vi "Value by Names.vi"(8 "error in (no error)":errorcluster, 10 "Children Names":string[](array[string]), 11 "OpenHW in":refnum<class "OpenHW.lvclass">) -> (0 "error out":errorcluster, 2 "HW Node":T1, 3 "OpenHW out":refnum<class "OpenHW.lvclass">)   [LabVIEW 2022 SP3, in "open-hw-mon-lv.lvlib" / "OpenHW.lvclass"]
uses:
  OpenHW.lvclass
  OpenHW.lvclass/OpenHW.ctl
  HW Node.ctl
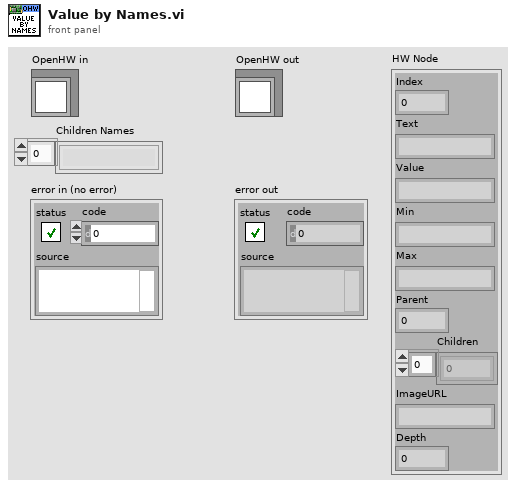
[diagram p1: front panel]
types:
  T1 = typedef "open-hw-mon-lv.lvlib/OpenHW.lvclass/HW Node.ctl" = cluster{"Index":i32, "Text":string, "Value":string, "Min":string, "Max":string, "Parent":i32, "Children":i32[], "ImageURL":string, "Depth":i32}
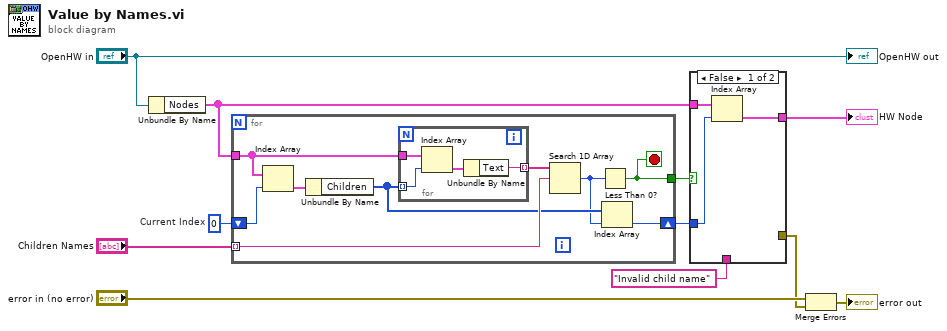
[diagram p0: block diagram]
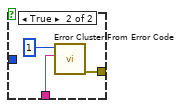
[diagram p2: hidden frame]
diagram:
  w10 = 0  # Current Index
  n1 = Unbundle By Name("OpenHW in") -> ("Nodes"=w7:T1[])
  n2 = for {
    tunnel: w7 -> [w18]
    shift-right: [w14] -> w8
    shift-left: w10 -> [w20]
    tunnel: [w12] -> w9
    tunnel: "Children Names" -> [w16] mode=indexing
    stop <- w12 stop-if-true
    n3 = Index Array(array=w18, index=w20) -> (element=w19:T1)
    n4 = Unbundle By Name(w19) -> ("Children"=w15:i32[])
    n5 = for {
      tunnel: w15 -> [w23] mode=indexing
      tunnel: w18 -> [w24]
      tunnel: [w21] -> w17 mode=indexing
      n6 = Index Array(array=w24, index=w23) -> (element=w22:T1)
      n7 = Unbundle By Name(w22) -> ("Text"=w21:string)
    }
    n8 = Search 1D Array(1D array=w17, element=w16) -> (index of element=w13:i32)  [unwired: 1 in]
    n9 = Less Than 0?(x=w13) -> (x < 0?=w12:bool)
    n10 = Index Array(array=w15, index=w13) -> (element=w14:i32)
  }
  n11 = case shown="False" w9 {
    tunnel: w8 -> [w26 _]
    tunnel: w7 -> [w27 _]
    tunnel: [w25 _] -> w4
    tunnel: "Invalid child name" -> [_ w29]
    tunnel: [_ w28] -> w2
    frame False {
      n12 = Index Array(array=w27, index=w26) -> (element=w25:T1)
    }
    frame True {
      n13 = call <vilib>:"Error Cluster From Error Code.vi"("error message (\"\")"=w29, "error code (0)"=1) -> ("error out"=w28:errorcluster)  [unwired: 7 in]
    }
  }
  "HW Node" <- w4
  n14 = Merge Errors("error in (no error)", w2) -> (→"error out":errorcluster)
  "OpenHW out" <- "OpenHW in"
